vi "dieukhienbangtay.vi"() -> ()   [LabVIEW 2019]
uses:
  <vilib>/Platform/TimedLoop/XDataNode/timing_clust.ctl
  <vilib>/Platform/TimedLoop/XDataNode/nitl_modes.ctl
  <vilib>/Platform/TimedLoop/XDataNode/wakeup.ctl
  <vilib>/platform/TimedLoop/XDataNode/XDataNode.xnode
  <vilib>/Platform/TimedLoop/XDataNode/XDNodeRunTimeDep.lvlib
panel:
  in  "TRAI":bool
  in  "PHAI":bool
  in  "LUI":bool
  in  "TIEN":bool
  in  "START":bool
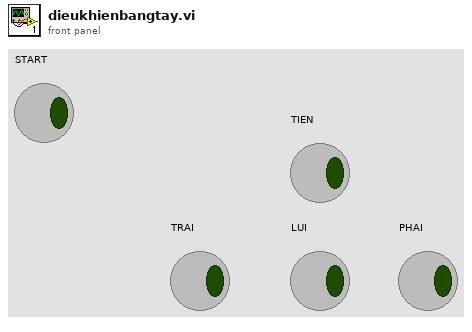
[diagram p1: front panel]
types:
  T1 = typedef "XDNodeRunTimeDep.lvlib/timing_clust.ctl" = cluster{"Expected End [f-1]":u64, "Actual End [f-1]":u64, "Finished Late? [f-1]":bool, "Expected End [i-1]":u64, "Actual End [i-1]":u64, "Finished Late? [i-1]":bool, "Expected Start [i]":u64, "Actual Start [i]":u64, "Expected Start [f]":u64, "Actual Start [f]":u64, "Source Name":string, "Structure Name":string, "Period":i64, "Deadline":i64, "Offset":i64, "Start":i64, "Priority":i32, "Timeout":i32, "Mode":T2, "Wakeup Reason":T3, "Error":errorcluster, "Source Type":string, "Secondary Source Type":string, "Global End Time":u64, "Global Start Time":u64, "Frame Duration":u64, "Iteration Duration":u64, "Assigned CPU":i32, "I/O Scan Engine Mode":u32}
  T2 = typedef "XDNodeRunTimeDep.lvlib/nitl_modes.ctl" = enum32{"No Change", "Process missed periods, maintain original phase", "Discard missed periods, maintain original phase", "Process missed periods, ignore original phase", "Discard missed periods, ignore original phase"}
  T3 = typedef "XDNodeRunTimeDep.lvlib/wakeup.ctl" = enum32{"Normal", "Aborted", "Asynchronous wakeup", "Timing source error", "Timed loop error", "Timeout"}
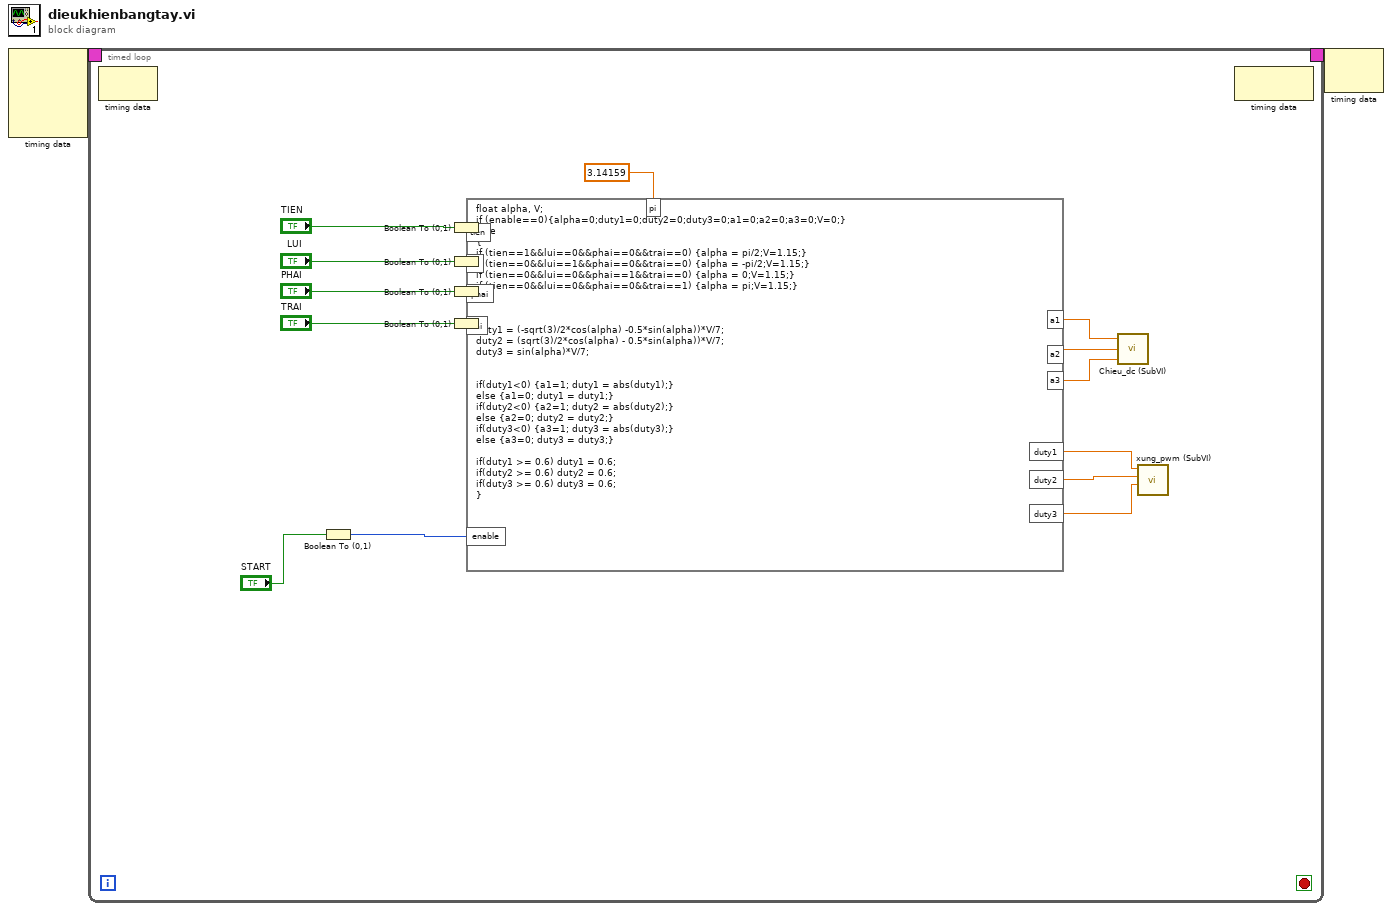
[diagram p0: block diagram]
diagram:
  n1 = node-c288() -> (w2:T1)  [unwired: 4 in]
  n2 = timed-loop {
    timing: w2 -> [_]
    timing-out: [_] -> w1
    stop <- _ stop-if-true
    n3 = node-c288() -> ()  [unwired: 1 in, 1 out]
    n4 = Boolean To (0,1)(Boolean="START") -> (0, 1=w18:i16)
    n5 = Boolean To (0,1)(Boolean="TIEN") -> (0, 1=w16:i16)
    n6 = Boolean To (0,1)(Boolean="LUI") -> (0, 1=w14:i16)
    n7 = Boolean To (0,1)(Boolean="PHAI") -> (0, 1=w12:i16)
    n8 = Boolean To (0,1)(Boolean="TRAI") -> (0, 1=w10:i16)
    n9 = formula code="float alpha, V;\nif (enable==0){alpha=0;duty1=0;duty2=0;duty3=0;a1=0;a2=0;a3=0;V=0;}\nelse\n{\nif (tien==1&&lui==0&&phai==0&&trai==0) {alpha = pi/2;V=1.15;}\nif (tien==0&&lui==1&&phai==0&&trai==0) {alpha = -pi/2;V=1.15;}\nif (tien==0&&lui==0&&phai==1&&trai==0) {alpha = 0;V=1.15;}\nif (tien==0&&lui==0&&phai==0&&trai==1) {alpha = pi;V=1.15;}\n\n\n\nduty1 = (-sqrt(3)/2*cos(alpha) -0.5*sin(alpha))*V/7;\nduty2 = (sqrt(3)/2*cos(alpha) - 0.5*sin(alpha))*V/7;\nduty3 = sin(alpha)*V/7;  \n\n\nif(duty1<0) {a1=1; duty1 = abs(duty1);}\nelse {a1=0; duty1 = duty1;}\nif(duty2<0) {a2=1; duty2 = abs(duty2);}\nelse {a2=0; duty2 = duty2;}\nif(duty3<0) {a3=1; duty3 = abs(duty3);}\nelse {a3=0; duty3 = duty3;}\n\nif(duty1 >= 0.6) duty1 = 0.6;\nif(duty2 >= 0.6) duty2 = 0.6;\nif(duty3 >= 0.6) duty3 = 0.6;\n}"("enable"=w18, "tien"=w16, "lui"=w14, "phai"=w12, "trai"=w10, "pi"=3.14159 ("input variable")) -> ("duty1"=w9:dbl, "duty2"=w8:dbl, "duty3"=w7:dbl, "a1"=w6:dbl, "a2"=w5:dbl, "a3"=w4:dbl)
    n10 = call "Chieu_dc (SubVI).vi"("a3"=w4, "a2"=w5, "a1"=w6) -> ()
    n11 = call "xung_pwm (SubVI).vi"("duty3 in"=w7, "duty2 in"=w8, "duty1 in"=w9) -> ()  [unwired: 6 in, 3 out]
    n12 = node-c288() -> ()  [unwired: 1 in, 1 out]
  }
  n13 = node-c288(w1) -> ()  [unwired: 1 out]
